vi "Request Elements.vi"(8 "error in (no error)":errorcluster, 11 "Event Response Handler in":refnum<class "Event Response Handler.lvclass">) -> (0 "error out":errorcluster, 3 "Event Response Handler out":refnum<class "Event Response Handler.lvclass">)   [LabVIEW 2020, in "Event Response Handler.lvclass"]
uses:
  Event Response Handler.lvclass
  Event Response Handler.lvclass/Event Response Handler.ctl
  Promises/Promise/Promise.lvclass
  ElementsValue/ElementsValue.lvclass
  Promises/Future/Future.lvclass
  ElementsValue/Some Fancy Data.ctl
panel:
  out "Value":T1
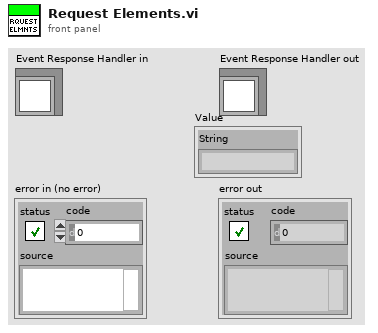
[diagram p1: front panel]
types:
  T1 = typedef "Futures-Examples.lvlib/ElementsValue.lvclass/Some Fancy Data.ctl" = cluster{"String":string}
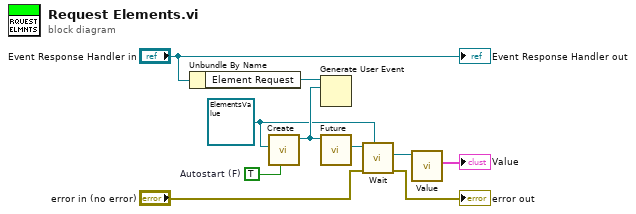
[diagram p0: block diagram]
diagram:
  w1 = refnum<class "ElementsValue.lvclass"> refnum ("Futures-Examples.lvlib:ElementsValue.lvclass")
  w8 = TRUE  # Autostart (F)
  n1 = Unbundle By Name("Event Response Handler in") -> ("Element Request"=w9:refnum<user-event>)
  n2 = call "Create.vi"("Autostart (F)"=w8, "Result Type (None)"=w1) -> ("Promise"=w7:refnum<class "Promise.lvclass">)  [unwired: 8 in, 1 out]
  n3 = Generate User Event(user event=w9, event data cluster=w7) -> ()  [unwired: 2 in, 2 out]
  n4 = call "Future.vi"("Promise in"=w7) -> ("Future"=w6:refnum<class "Future.lvclass">)  [unwired: 9 in, 1 out]
  n5 = call "Wait.vi"("Result Type (None)"=w1, "error in (no error)"="error in (no error)", "Future in"=w6) -> ("error out"=→"error out":errorcluster, "Result"=w5:refnum<class>)  [unwired: 7 in]
  n6 = call "Value.vi"("ElementsValue in"=w5) -> ("Value"=→"Value":T1)  [unwired: 10 in]
  "Event Response Handler out" <- "Event Response Handler in"
